vi "TR_JoystickStatus.vi"(11 "Mouse in":refnum<class "Joystick.lvclass">) -> ()   [LabVIEW 2021, in "InputDevice.lvlib" / "Joystick.lvclass"]
uses:
  Joystick.lvclass
  eb7bb245-cb1a-4027-9ed5-b4438251725f.vi
  4b2ba3d0-6e9e-49b1-aade-53c9626005bb.vi
  8ae88d8c-86e8-4183-9e02-5cb064982b42.vi
  <vilib>/Utility/inputDevices.llb/joystickAcquire.vi
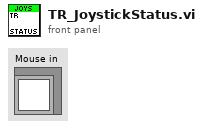
[diagram p1: front panel]
types:
  T1 = typedef "Joystick.lvclass/data.ctl" = cluster{"DeviceID":refnum<k1>, "JoyButtonInfo":refnum<user-event>, "JoyAxisInfo":refnum<user-event>, "JoyDirectionInfo":refnum<user-event>, "Joystick":refnum<event-registration>, "StopNotifier":refnum<notifier>}
  T2 = cluster{"X axis":i32, "Y axis":i32, "Z axis":i32, "X axis rotation":i32, "Y axis rotation":i32, "Z axis rotation":i32, "U axis":i32, "V axis":i32}
  T3 = cluster{"button 1":bool, "button 2":bool, "button 3":bool, "button 4":bool, "button 5":bool, "button 6":bool, "button 7":bool, "button 8":bool, "button 9":bool, "button 10":bool, "button 11":bool, "button 12":bool, "button 13":bool, "button 14":bool, "button 15":bool, "button 16":bool, "button 17":bool, "button 18":bool, "button 19":bool, "button 20":bool, "button 21":bool, "button 22":bool, "button 23":bool, "button 24":bool, "button 25":bool, "button 26":bool, "button 27":bool, "button 28":bool, "button 29":bool, "button 30":bool, "button 31":bool, "button 32":bool}
  T4 = cluster{"pov 1":i32, "pov 2":i32, "pov 3":i32, "pov 4":i32}
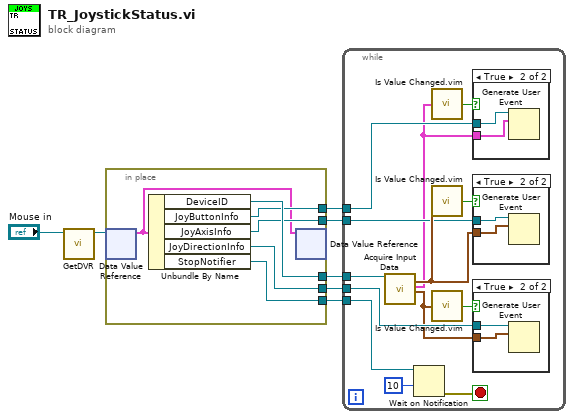
[diagram p0: block diagram]
diagram:
  n1 = call "GetDVR.vi"("Mouse"="Mouse in") -> ("DVR"=w6:refnum<data-value>)  [unwired: 9 in, 1 out]
  n2 = in-place {
    in-place-border: [w13] -> w5
    in-place-border: [w12] -> w4
    in-place-border: [w11] -> w3
    in-place-border: [w10] -> w2
    in-place-border: [w8] -> w1
    n3 = in-place-dvr #1(w6) -> (w9:T1)  [unwired: 1 out]
    n4 = Unbundle By Name(w9) -> ("DeviceID"=w13:refnum<k1>, "JoyButtonInfo"=w12:refnum<user-event>, "JoyAxisInfo"=w11:refnum<user-event>, "JoyDirectionInfo"=w8:refnum<user-event>, "StopNotifier"=w10:refnum<notifier>)
    n5 = in-place-dvr #1(w9) -> ()  [unwired: 2 out]
  }
  n6 = while {
    tunnel: w5 -> [w26]
    tunnel: w4 -> [w17]
    tunnel: w3 -> [w18]
    tunnel: w2 -> [w21]
    tunnel: w1 -> [w19]
    stop <- w22 stop-if-true
    n7 = call-poly <vilib>:"Acquire Input Data.vi"("device ID"=w26) -> ("axis info"=w24:T2, "button info"=w14:T3, "direction info"=w15:T4)  [unwired: 14 in, 2 out]
    n8 = Wait on Notification(notifier=w21, timeout in ms (-1)=10) -> (error out=w22:errorcluster)  [unwired: 2 in, 3 out]
    n9 = call "Is Value Changed.vim"("value"=w14) -> ("changed or first call?"=w16:bool)
    n10 = call "Is Value Changed.vim"("value"=w24) -> ("changed or first call?"=w25:bool)
    n11 = call "Is Value Changed.vim"("value"=w15) -> ("changed or first call?"=w23:bool)
    n12 = case shown="True" w16 {
      tunnel: w17 -> [_ w28]
      tunnel: w14 -> [_ w27]
      frame False {
      }
      frame True {
        n13 = Generate User Event(user event=w28, event data cluster=w27) -> ()  [unwired: 2 in, 2 out]
      }
    }
    n14 = case shown="True" w25 {
      tunnel: w18 -> [_ w32]
      tunnel: w24 -> [_ w31]
      frame False {
      }
      frame True {
        n15 = Generate User Event(user event=w32, event data cluster=w31) -> ()  [unwired: 2 in, 2 out]
      }
    }
    n16 = case shown="True" w23 {
      tunnel: w19 -> [_ w30]
      tunnel: w15 -> [_ w29]
      frame False {
      }
      frame True {
        n17 = Generate User Event(user event=w30, event data cluster=w29) -> ()  [unwired: 2 in, 2 out]
      }
    }
  }
